vi "Test Helper Loop Broadcast Stopped State.vi"(8 "error in (no error)":errorcluster, 11 "Helper Loop Test In":refnum<class "Helper Loop Test.lvclass">) -> (0 "error out":errorcluster, 3 "Helper Loop Test Out":refnum<class "Helper Loop Test.lvclass">)   [LabVIEW 2020, in "Helper Loop Test.lvclass"]
uses:
  Helper Loop Test.lvclass
  C:/Program Files (x86)/National Instruments/LabVIEW 2020/vi.lib/Astemes/LUnit/Test Case.lvclass
  source/Framework Test Suite/Mock Process/Mock Process.lvclass
  C:/git/astemes-triarc-framework/source/Framework/Process/Process.lvclass
  source/Framework/Process/Process.lvclass/Process.ctl
  <vilib>/Astemes/LUnit/Test Case.lvclass/Test Case.ctl
  5bd70ed2-b5d4-4798-a2af-26ca39621187.vi
  source/Framework/Process/Public/Lifecycle/Get Lifecycle State.vi
  <vilib>/Astemes/LUnit/Append Pass Result.vi
  <vilib>/Astemes/LUnit/Append Fail Result.vi
  source/Framework/Broadcast Event Helpers/Execution timer.vi
  source/Framework/Process/Private/SubVIs/Wait for finish.vi
  source/Framework/Process/Private/SubVIs/Set Lifecycle State.vi
  source/Framework/Process/Protected/Messaging/Send Message.vi
  <vilib>/Astemes/LUnit/Describe Comparison.vi
  <vilib>/Astemes/LUnit/Compare Variants.vi
  <vilib>/Utility/error.llb/Clear Errors.vi
  source/Framework/Process/Private/SubVIs/Handle Debug Data.vi
  <vilib>/Astemes/LUnit/Variant to string.vi
  source/Framework/Logging/Log Debug.vi
  <vilib>/AdvancedString/1D String Array to Delimited String.vi
  <vilib>/Utility/High Resolution Relative Seconds.vi
  <vilib>/Utility/error.llb/Error Cluster From Error Code.vi
  source/Framework/Broadcast Event Dequeuers/Dequeue Broadcast Message.vi
  source/Framework/Process/Public/Read Name.vi
  <vilib>/Utility/Data Type/Get Type Information.vi
  <vilib>/Utility/LVClass/Get LV Class Name.vi
  source/Framework/Callback/Callback.lvclass
  source/Framework/Process/Process.lvclass
  Helper Loop Test.lvclass/Helper Loop Test.ctl
  <vilib>/Astemes/LUnit/Test Case.lvclass
  source/Framework/Broadcast Event Dequeuers/Broadcast Event Dequeuers.lvlib
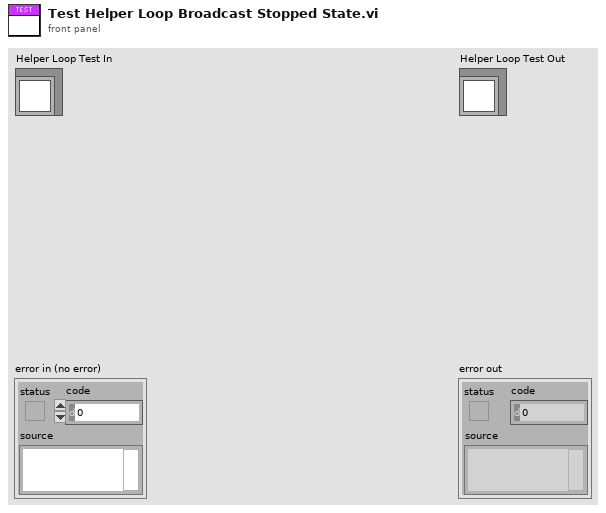
[diagram p1: front panel]
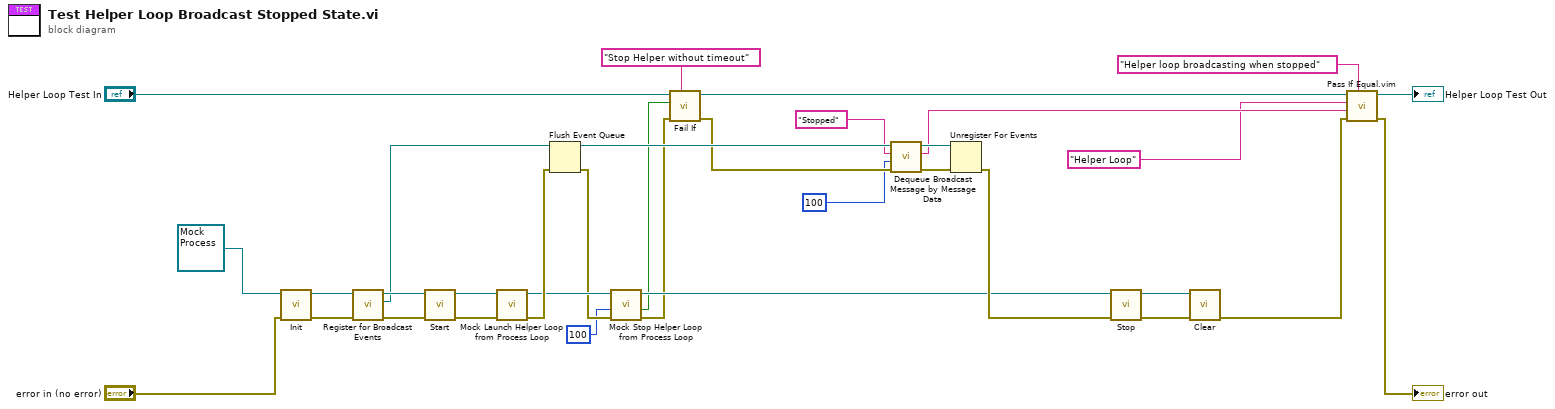
[diagram p0: block diagram]
diagram:
  n1 = call-dynamic "Init.vi"("error in (no error)"="error in (no error)", "Mock Process In"=refnum<class "Mock Process.lvclass"> refnum) -> ("error out"=w32:errorcluster, "Mock Process Out"=w33:refnum<class "Mock Process.lvclass">)  [unwired: 8 in]
  n2 = call "Register for Broadcast Events.vi"("error in (no error)"=w32, "Process In"=w33) -> ("error out"=w30:errorcluster, "Event Registration Refnum Out"=w20:refnum<event-registration>, "Process Out"=w31:refnum<class "Mock Process.lvclass">)  [unwired: 7 in]
  n3 = call "Start.vi"("error in (no error)"=w30, "Process In"=w31) -> ("error out"=w28:errorcluster, "Process Out"=w29:refnum<class "Mock Process.lvclass">)  [unwired: 7 in, 1 out]
  n4 = call "Mock Launch Helper Loop from Process Loop.vi"("error in (no error)"=w28, "Mock Process in"=w29) -> ("error out"=w16:errorcluster, "Mock Process out"=w15:refnum<class "Mock Process.lvclass">)  [unwired: 8 in]
  n5 = Flush Event Queue(0:w20, 3:w16) -> (8:w17:refnum<event-registration>, 11:w13:errorcluster)  [unwired: 4 in, 1 out]
  n6 = call "Mock Stop Helper Loop from Process Loop.vi"("error in (no error)"=w13, "timeout in ms (-1)"=100, "Mock Process in"=w15) -> ("error out"=w10:errorcluster, "timed out?"=w8:bool, "Mock Process out"=w14:refnum<class "Mock Process.lvclass">)  [unwired: 6 in]
  n7 = call <vilib>:"Fail If.vi"("Description"="Stop Helper without timeout", "error in (no error)"=w10, "Fail?"=w8, "LUnit Test Case In"="Helper Loop Test In") -> ("error out"=w9:errorcluster, "LUnit Test Case Out"=w11:refnum<class "Helper Loop Test.lvclass">)  [unwired: 6 in]
  n8 = call "Dequeue Broadcast Message by Message Data.vi"("error in (no error)"=w9, "Timeout (-1)"=100, "Message Data"="Stopped" ("y"), "Event Registration Refnum"=w17) -> ("error out"=w6:errorcluster, "Message"=w2:string, "Event Registration Refnum Out"=w19:refnum<event-registration>)  [unwired: 3 in, 2 out]
  n9 = Unregister For Events(event registration refnum=w19, error in=w6) -> (error out=w18:errorcluster)
  n10 = call "Stop.vi"("error in (no error)"=w18, "Process In"=w14) -> ("error out"=w27:errorcluster, "Process Out"=w3:refnum<class "Mock Process.lvclass">)  [unwired: 7 in, 1 out]
  n11 = call-dynamic "Clear.vi"("error in (no error)"=w27, "Mock Process In"=w3) -> ("error out"=w26:errorcluster)  [unwired: 9 in]
  n12 = call "Pass If Equal.vim"("Description"="Helper loop broadcasting when stopped", "error in (no error)"=w26, "Actual"=w2, "Expected"="Helper Loop" ("y"), "LUnit Test Case In"=w11) -> ("error out"=→"error out":errorcluster, "LUnit Test Case Out"=→"Helper Loop Test Out":refnum<class "Helper Loop Test.lvclass">)  [unwired: 5 in]
